vi "Move2Vector.vi"(8 "Motor Speed":u16(ring)=30000 items=["SLOW"=3300, "MEDIUM"=30000, "FAST"=65000], 10 "Angle":dbl, 11 "XY Vector":dbl[](array[numeric])) -> (2 "Finished?":bool)   [LabVIEW 2015]
uses:
  LabVIEW for ezAFM/LV-PGC 2019-05a/In Progress/ezAFM LabVIEW/NMI coordinates.ctl
  D:/LabVIEW for ezAFM/LV-PGC 2019-05a/Special Equipment/ezAFM/NMI Integration Code/ezCommander.dll
  LabVIEW for ezAFM/LV-PGC 2019-05a/Special Equipment/ezAFM/NMI Integration Code/ezCommander.dll
panel:
  out "Coordinate System Diagram":T1={"OK"=TRUE}
  # "CAD Cartesian Layout"
  # "+x"
  # "+y"
  # "IMAQ Pixel Coordinates"
  # "+x"
  # "0,0"
  # "+y"
  # "ezAFM Coordinates"
  # "+y"
  # "ezAFM coordinates are \nexactly the negative of\nXY values in CAD design"
  # "+x"
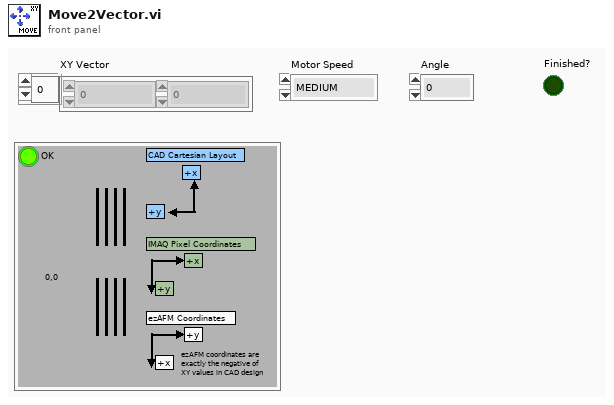
[diagram p1: front panel]
types:
  T1 = typedef "NMI coordinates.ctl" = cluster{"OK":bool}
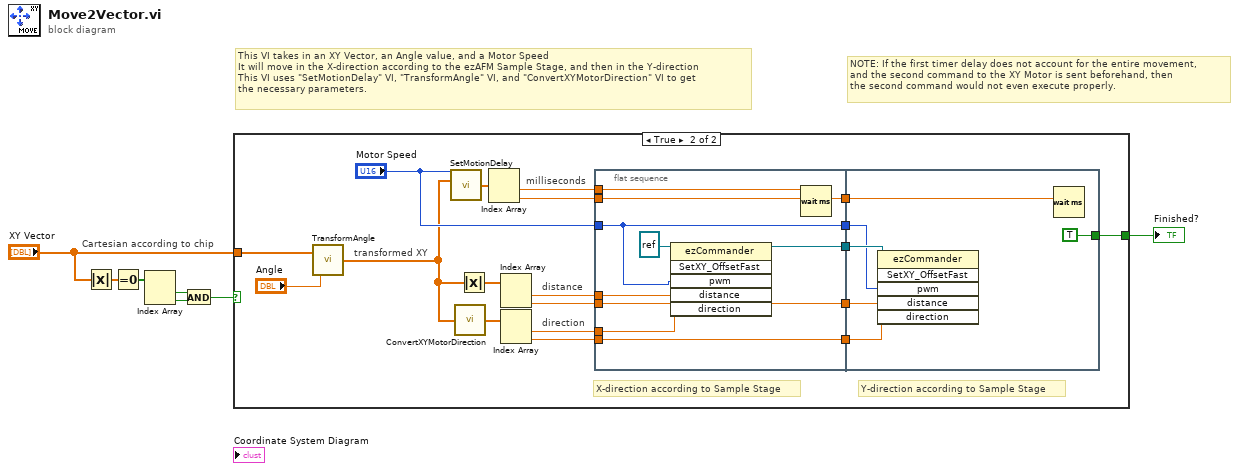
[diagram p0: block diagram]
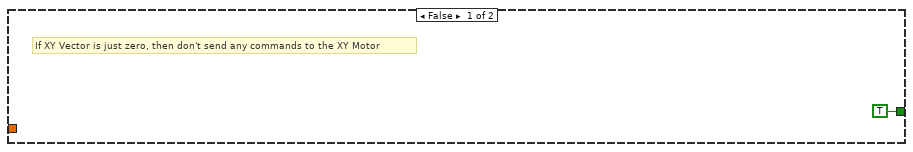
[diagram p2: hidden frame]
diagram:
  # "Cartesian according to chip"
  # "NOTE: If the first timer delay does not account for the entire movement,\nand the second command to the XY Motor is sent beforehand, then\nthe second command would not even execute properly."
  # "This VI takes in an XY Vector, an Angle value, and a Motor Speed\nIt will move in the X-direction according to the ezAFM Sample Stage, and then in the Y-direction\nThis VI uses \"SetMotionDelay\" VI, \"TransformAngle\" VI, and \"ConvertXYMotorDirection\" VI to get \nthe necessary parameters."
  n1 = Absolute Value(x="XY Vector") -> (abs(x)=w6:dbl[])
  n2 = Equal To 0?(x=w6) -> (x = 0?=w5:bool[])
  n3 = Index Array(array=w5) -> (element #1=w4:bool, element #2=w3:bool)  [unwired: 2 in]
  n4 = And(x=w4, y=w3) -> (x .and. y?=w2:bool)
  n5 = case shown="True" w2 {
    tunnel: [TRUE ("Finished?") w10] -> w7
    tunnel: "XY Vector" -> [_ w9]
    frame False {
      # "If XY Vector is just zero, then don't send any commands to the XY Motor"
    }
    frame True {
      # "direction"
      # "distance"
      # "transformed XY"
      # "milliseconds"
      # "Y-direction according to Sample Stage"
      # "X-direction according to Sample Stage"
      n6 = call "TransformAngle.vi"("Angle"="Angle", "XY Vector"=w9) -> ("Result Vector"=w11:dbl[])
      n7 = call "SetMotionDelay.vi"("Motor Speed"="Motor Speed", "XY Vector"=w11) -> ("Delays"=w21:dbl[])
      n8 = call "ConvertXYMotorDirection.vi"("XY Vector"=w11) -> ("XY Motor Directions"=w18:dbl[])
      n9 = Absolute Value(x=w11) -> (abs(x)=w12:dbl[])
      n10 = Index Array(array=w21) -> (element #1=w20:dbl, element #2=w19:dbl)  [unwired: 2 in]
      n11 = Index Array(array=w12) -> (element #1=w15:dbl, element #2=w14:dbl)  [unwired: 2 in]
      n12 = Index Array(array=w18) -> (element #1=w17:dbl, element #2=w16:dbl)  [unwired: 2 in]
      n13 = flat-sequence {
        tunnel: [w35] -> w27
        tunnel: w20 -> [w34]
        tunnel: [w33] -> w26
        tunnel: w19 -> [w33]
        tunnel: w17 -> [w31]
        tunnel: [w32] -> w25
        tunnel: w16 -> [w32]
        tunnel: w15 -> [w30]
        tunnel: [w29] -> w24
        tunnel: w14 -> [w29]
        tunnel: "Motor Speed" -> [w28]
        tunnel: [w28] -> w23
        tunnel: w27 -> [w42]
        tunnel: w26 -> [w41]
        tunnel: w25 -> [w40]
        tunnel: w24 -> [w39]
        tunnel: w23 -> [w38]
        tunnel: [TRUE ("Finished?")] -> w10
        frame #0 {
          n14 = invoke class="ezCommander" method="SetXY_OffsetFast"(reference=refnum<k24> refnum ("ezAFM Ref"), "pwm"=w28, "distance"=w30, "direction"=w31) -> (reference out=w35:refnum<k24>)  [unwired: 2 in, 5 out]
          n15 = Wait (ms)(milliseconds to wait=w34) -> ()  [unwired: 1 out]
        }
        frame #1 {
          n16 = invoke class="ezCommander" method="SetXY_OffsetFast"(reference=w42, "pwm"=w38, "distance"=w39, "direction"=w40) -> ()  [unwired: 2 in, 6 out]
          n17 = Wait (ms)(milliseconds to wait=w41) -> ()  [unwired: 1 out]
        }
      }
    }
  }
  "Finished?" <- w7
